vi "Get_Current_Scan_server.vi"(0 "Desired Channels":string[](array[string])) -> (1 "Ch Description Array":T1[](array[typedef]) {"Duty" format="%.0b"; "D" format="%#_5g"; "C" format="%#_5g"; "B" format="%#_5g"; "A" format="%#_5g"}, 2 "String values":string[](array[string]), 3 "Numerical Values":dbl[](array[numeric]) format="%.2f")   [LabVIEW 2012]
uses:
  ADAM Client/Sub VIs/ADAM Controls/Ch_description_ADAM.ctl
  ADAM Client/Sub VIs/ADAM Controls/Module_type_ADAM.ctl
  ADAM Client/Sub VIs/ADAM Controls/Function_ADAM.ctl
  ADAM Client/Sub VIs/ADAM Controls/Channel_State.ctl
  ADAM Client/Sub VIs/ADAM Controls/Calib_type_ADAM.ctl
  ADAM Client/Sub VIs/ADAM Controls/Address.ctl
  ADAM_Global.vi
  Sub VI's/Channel_Description_Global.vi
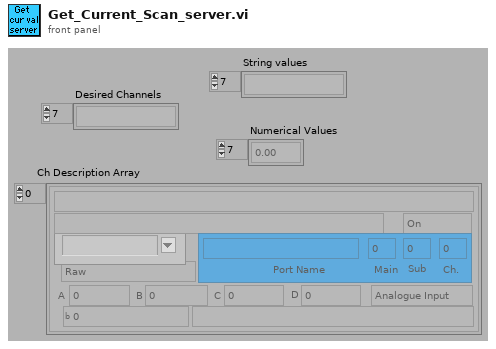
[diagram p1: front panel]
types:
  T1 = typedef "Ch_description_ADAM.ctl" = cluster{"Ch Name":string, "Type":T2, "Function":T3, "Ch State":T4, "Calibration type":T5, "A":dbl, "B":dbl, "C":dbl, "D":dbl, "Comments":string, "Address":T6, "String":string, "Duty":u16}
  T2 = typedef "Module_type_ADAM.ctl" = string
  T3 = typedef "Function_ADAM.ctl" = enum16{"Analogue Input", "Digital Input", "Event counter", "Event rate", "Analogue Output", "Digital Output", "Relay Output"}
  T4 = typedef "Channel_State.ctl" = enum16{"On", "Off", "Always On", "Always Off"}
  T5 = typedef "Calib_type_ADAM.ctl" = enum16{"Raw", "Bx + A", "Cx^2 + Bx + A", "Dx^3 + Cx^2 + Bx + A", "In Band", "Hi-Tec Q", "Hi-Tec M_dot", "Text"}
  T6 = typedef "Address.ctl" = cluster{"Main":i32, "Ch.":i32, "Sub":i32, "Port Name":string}
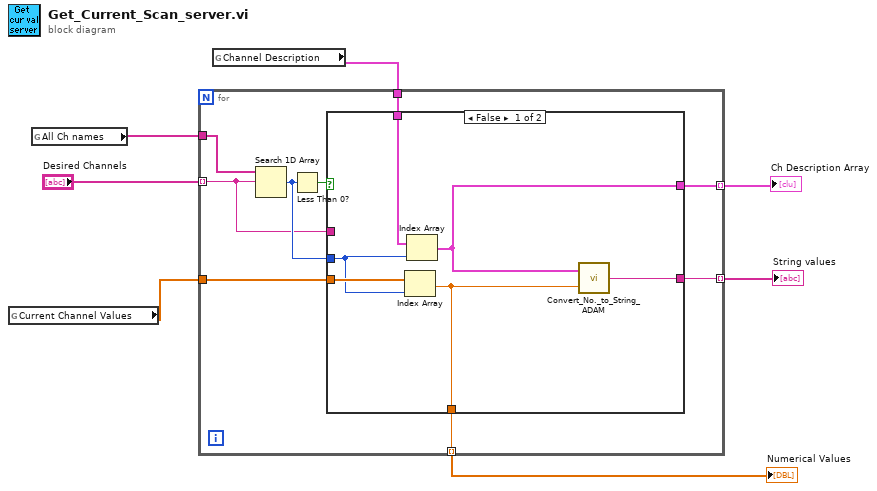
[diagram p0: block diagram]
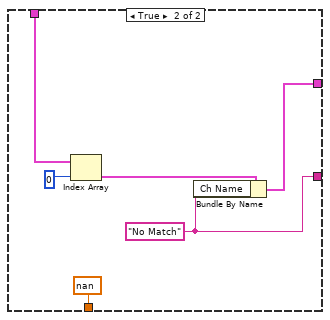
[diagram p2: hidden frame]
diagram:
  n1 = global read "ADAM_Global.vi" "Current Channel Values"() -> (w6:dbl[])
  n2 = global read "ADAM_Global.vi" "All Ch names"() -> (w7:string[])
  n3 = global read "Channel_Description_Global.vi" "Channel Description"() -> (w1:T1[])
  n4 = for {
    tunnel: "Desired Channels" -> [w8] mode=indexing
    tunnel: w7 -> [w16]
    tunnel: [w14] -> w5 mode=indexing
    tunnel: w6 -> [w12]
    tunnel: w1 -> [w11]
    tunnel: [w10] -> w4 mode=indexing
    tunnel: [w9] -> w2 mode=indexing
    n5 = Search 1D Array(1D array=w16, element=w8) -> (index of element=w13:i32)  [unwired: 1 out]
    n6 = Less Than 0?(x=w13) -> (x < 0?=w15:bool)
    n7 = case shown="False" w15 {
      tunnel: [w20 w24] -> w14
      tunnel: w13 -> [w18 _]
      tunnel: w12 -> [w22 _]
      tunnel: w11 -> [w21 w27]
      tunnel: [w19 nan] -> w10
      tunnel: [w17 w25] -> w9
      tunnel: w8 -> [_ _]
      frame False {
        n8 = Index Array(array=w22, index=w18) -> (element=w19:dbl)
        n9 = Index Array(array=w21, index=w18) -> (element=w17:T1)
        n10 = call "Convert_No._to_String_ADAM.vi"("Input number"=w19, "Ch Description"=w17) -> ("Output sting"=w20:string)
      }
      frame True {
        w24 = "No Match"
        n11 = Index Array(array=w27, index=0 ("Index")) -> (element=w26:T1)
        n12 = Bundle By Name(cluster=w26, "Ch Name"=w24) -> (w25:T1)
      }
    }
  }
  "String values" <- w5
  "Numerical Values" <- w4
  "Ch Description Array" <- w2
